vi "Launcher.vi"() -> ()   [LabVIEW 2020, in "DAQ.lvlib"]
uses:
  DAQ_Base_class/subvi/DAQ.lvlib
  DAQ_Base_class/DAQ_Base.lvclass
panel:
  out "Stop":bool
  in  "CollectorChannelEnable":bool[](array[boolean])
  out "自动采集第2段":dbl[][](graph)
  out "自动采集第1段":dbl[][](graph)
  out "手动采集":dbl[][](graph)
  in  "停止":bool
  out "RealTimeValue":dbl[](array[numeric])
  # "SMO架构暂时用不到"
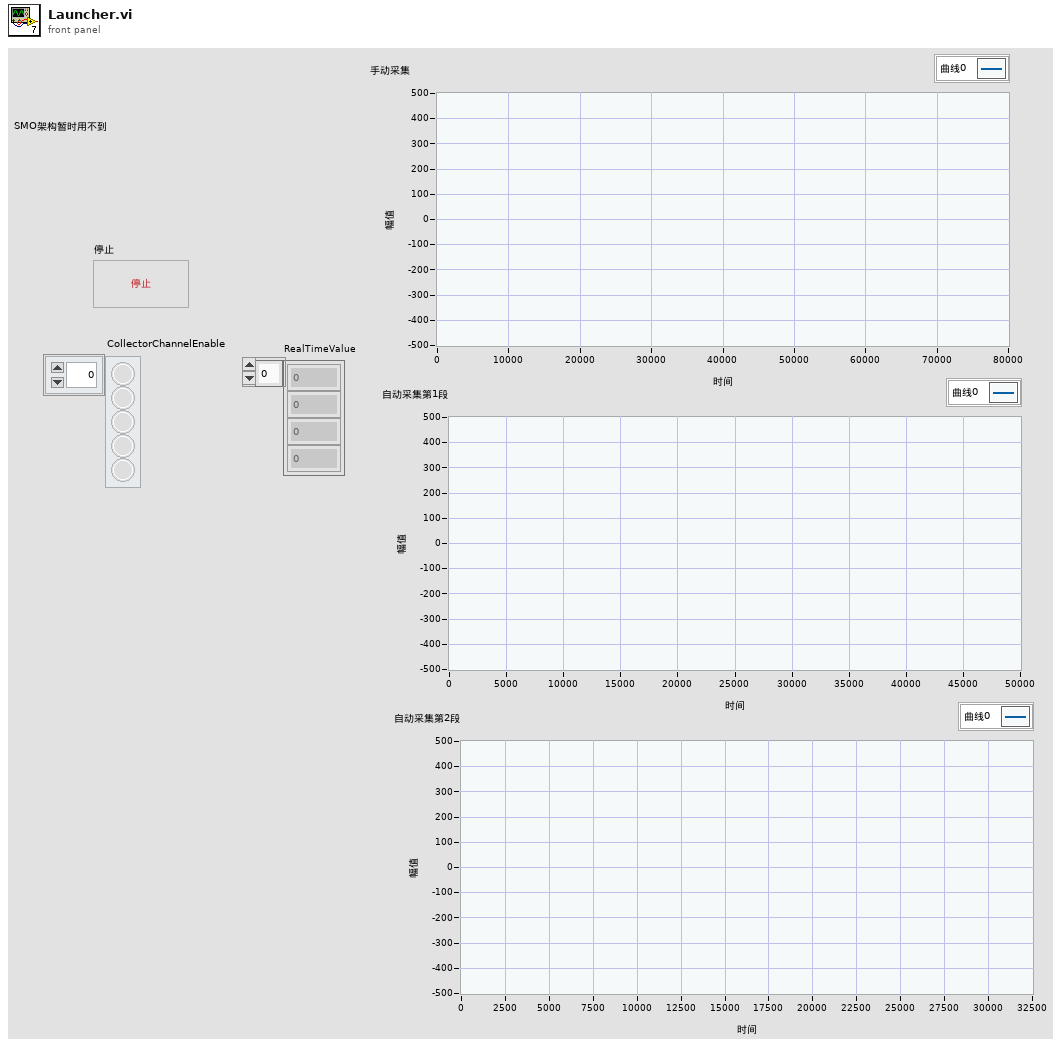
[diagram p1: front panel]
types:
  T1 = typedef "DAQ.lvlib/DAQ_Base.lvclass/DataCollector.ctl" = cluster{"DataCollectArry":dbl[][], "Update":bool}
  T2 = cluster{"CollectDataQueue":refnum<queue>, "ArryDataCollectorChannel":T1[], "RealTimeValues":dbl[]}
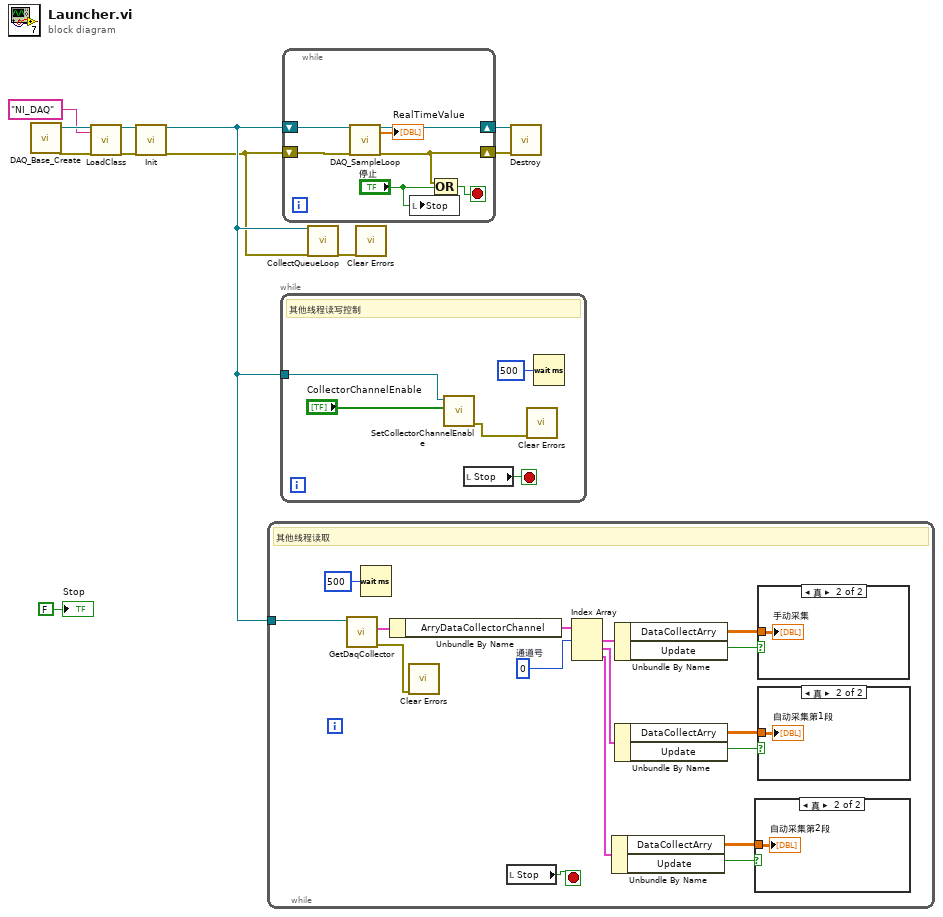
[diagram p0: block diagram]
diagram:
  n1 = call "DAQ_Base_Create.vi"() -> ("reference out"=w11:refnum<class "DAQ_Base.lvclass">, "error out"=w10:errorcluster)  [unwired: 18 in]
  n2 = call "LoadClass.vi"("reference in"=w11, "ClassName"="NI_DAQ", "error in (no error)"=w10) -> ("reference out"=w5:refnum<class "DAQ_Base.lvclass">, "error out"=w4:errorcluster)  [unwired: 15 in]
  n3 = call-dynamic "Init.vi"("reference in"=w5, "error in (no error)"=w4) -> ("reference out"=w3:refnum<class "DAQ_Base.lvclass">, "error out"=w2:errorcluster)  [unwired: 16 in]
  n4 = while {
    tunnel: w3 -> [w26]
    stop <- w12 stop-if-true
    w20 = 0  # 通道号
    # "其他线程读取"
    n5 = call-dynamic "GetDaqCollector.vi"("reference in"=w26) -> ("error out"=w13:errorcluster, "DaqCollector"=w25:T2)  [unwired: 8 in, 1 out]
    n6 = Wait (ms)(milliseconds to wait=u32 500 ("等待时间（毫秒）")) -> ()  [unwired: 1 out]
    n7 = Unbundle By Name(w25) -> ("ArryDataCollectorChannel"=w24:T1[])
    n8 = call <vilib>:"Clear Errors.vi"("error in (no error)"=w13) -> ()  [unwired: 5 in, 2 out]
    n9 = local read "Stop"() -> (w12:bool)
    n10 = Index Array(array=w24, index #1=w20) -> (element #1=w23:T1, element #2=w15:T1, element #3=w14:T1)  [unwired: 2 in]
    n11 = Unbundle By Name(w14) -> ("DataCollectArry"=w16:dbl[][], "Update"=w17:bool)
    n12 = Unbundle By Name(w23) -> ("DataCollectArry"=w21:dbl[][], "Update"=w22:bool)
    n13 = Unbundle By Name(w15) -> ("DataCollectArry"=w19:dbl[][], "Update"=w18:bool)
    n14 = case shown="真" w17 {
      tunnel: w16 -> [_ w28]
      frame False {
      }
      frame True {
        "自动采集第2段" <- w28
      }
    }
    n15 = case shown="真" w22 {
      tunnel: w21 -> [_ w30]
      frame False {
      }
      frame True {
        "手动采集" <- w30
      }
    }
    n16 = case shown="真" w18 {
      tunnel: w19 -> [_ w29]
      frame False {
      }
      frame True {
        "自动采集第1段" <- w29
      }
    }
  }
  n17 = while {
    tunnel: w3 -> [w34]
    stop <- w31 stop-if-true
    # "其他线程读写控制"
    n18 = call-dynamic "SetCollectorChannelEnable.vi"("CollectorChannelEnable"="CollectorChannelEnable", "reference in"=w34) -> ("error out"=w32:errorcluster)  [unwired: 8 in, 1 out]
    n19 = local read "Stop"() -> (w31:bool)
    n20 = call <vilib>:"Clear Errors.vi"("error in (no error)"=w32) -> ()  [unwired: 5 in, 2 out]
    n21 = Wait (ms)(milliseconds to wait=u32 500 ("等待时间（毫秒）")) -> ()  [unwired: 1 out]
  }
  n22 = while {
    shift-right: [w42] -> w9
    shift-left: w3 -> [w41]
    shift-right: [w38] -> w8
    shift-left: w2 -> [w40]
    stop <- w39 stop-if-true
    n23 = call-dynamic "DAQ_SampleLoop.vi"("reference in"=w41, "error in (no error)"=w40) -> ("reference out"=w42:refnum<class "DAQ_Base.lvclass">, "RealTimeValue"=→"RealTimeValue":dbl[], "error out"=w38:errorcluster)  [unwired: 15 in]
    n24 = local write "Stop"("停止") -> ()
    n25 = Compound Arithmetic op=OR ("复合运算")(w38, "停止") -> (w39:bool)
  }
  n26 = call-dynamic "CollectQueueLoop.vi"("reference in"=w3, "error in (no error)"=w2) -> ("error out"=w6:errorcluster)  [unwired: 16 in, 1 out]
  n27 = call <vilib>:"Clear Errors.vi"("error in (no error)"=w6) -> ()  [unwired: 5 in, 2 out]
  n28 = call-dynamic "Destroy.vi"("reference in"=w9, "error in (no error)"=w8) -> ()  [unwired: 16 in, 2 out]
  "Stop" <- FALSE ("Stop")
